vi "MGCC_BlkStart_Globals.vi"() -> ()   [LabVIEW 2016]
panel:
  out "BlackStartCmd":bool[](array[boolean])
  out "BlackStartSuccess":bool[](array[boolean])
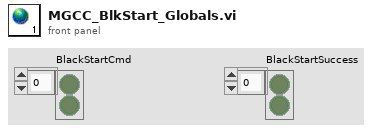
[diagram p1: front panel]
diagram:
